vi "GetAbsoluteAngle.vi"(8 "error in (no error)":errorcluster, 11 "Angle in":refnum<class "Angle.lvclass">) -> (0 "error out":errorcluster, 2 "Absolute angle (Deg.)":dbl)   [LabVIEW 2013, in "Angle.lvclass"]
doc: "Takes an angle input and returns the absolute angle in degrees as a double."
uses:
  Angle.lvclass
  Angle.lvclass/Angle.ctl
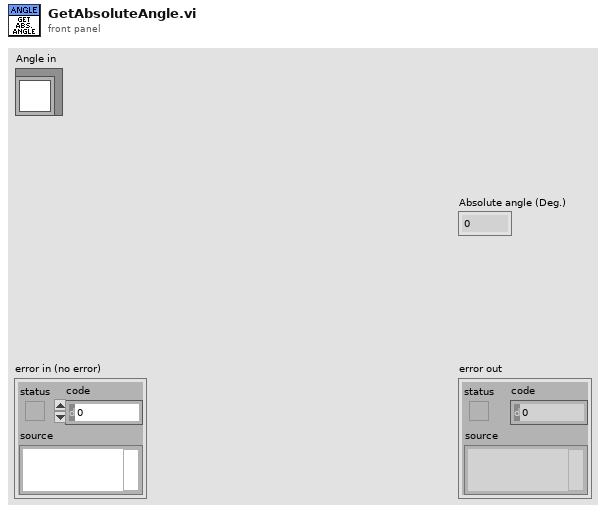
[diagram p1: front panel]
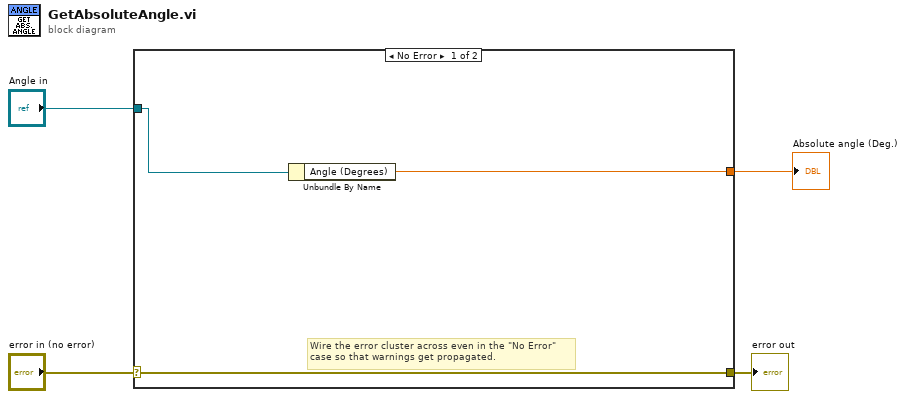
[diagram p0: block diagram]
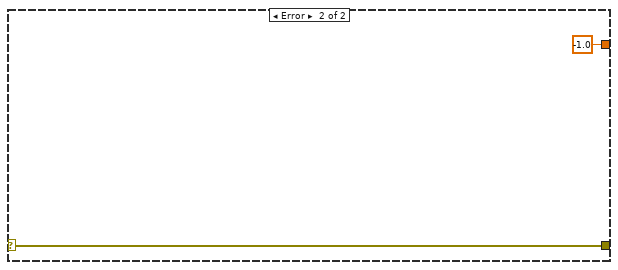
[diagram p2: hidden frame]
diagram:
  n1 = case shown="No Error" "error in (no error)" {
    selector: "error in (no error)" -> [w7 w9]
    tunnel: [w7 w9] -> w3
    tunnel: "Angle in" -> [w6 _]
    tunnel: [w5 -1.0 ("Angle (Degrees)")] -> w1
    frame No Error {
      # "Wire the error cluster across even in the \"No Error\"\ncase so that warnings get propagated."
      n2 = Unbundle By Name(w6) -> ("Angle (Degrees)"=w5:dbl)
    }
    frame Error {
    }
  }
  "error out" <- w3
  "Absolute angle (Deg.)" <- w1
